vi "Path Is Funnel.vi"(1 "Path Information":T2) -> (0 "Is Funnel?":bool)   [LabVIEW 2013]
doc: "This VI determines whether or not a path is actually a funnel. It must have two curves (C's) and if it has a line (L), the last point must be the same as the starting point."
uses:
  <vilib>/Analysis/Matrix/Datatypes/RealMatrix.ctl
  <vilib>/Analysis/Matrix/NI_Matrix.lvlib
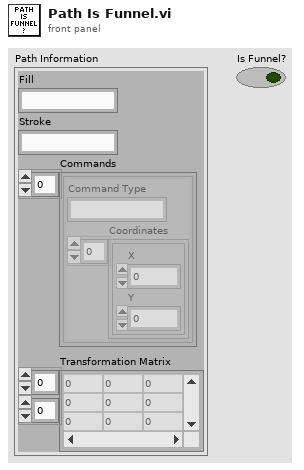
[diagram p1: front panel]
types:
  T1 = typedef "NI_Matrix.lvlib/RealMatrix.ctl" = dbl[][]
  T2 = cluster{"Fill":string, "Stroke":string, "Commands":cluster{"Command Type":string, "Coordinates":cluster{"X":dbl, "Y":dbl}[]}[], "Transformation Matrix":T1}
  T3 = cluster{"Command Type":string, "Coordinates":cluster{"X":dbl, "Y":dbl}[]}[]
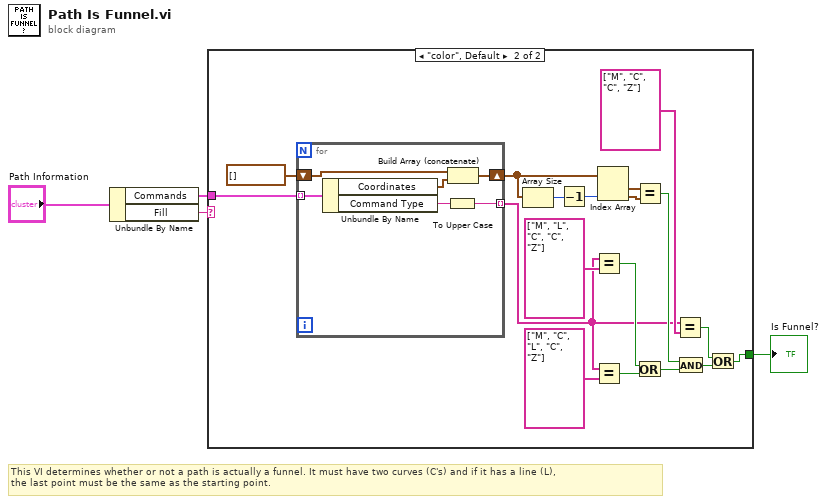
[diagram p0: block diagram]
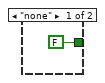
[diagram p2: hidden frame]
diagram:
  # "This VI determines whether or not a path is actually a funnel. It must have two curves (C's) and if it has a line (L),\nthe last point must be the same as the starting point."
  n1 = Unbundle By Name("Path Information") -> ("Commands"=w3:T3, "Fill"=w4:string)
  n2 = case shown="\"color\", Default" w4 {
    tunnel: w3 -> [_ w7]
    tunnel: [FALSE w6] -> w1
    frame "none" {
    }
    frame "color", Default {
      n3 = for {
        tunnel: w7 -> [w29] mode=indexing
        tunnel: [w24] -> w8 mode=indexing
        shift-right: [w27] -> w13
        shift-left: cluster{"X":dbl, "Y":dbl}[] [] -> [w28]
        n4 = Unbundle By Name(w29) -> ("Coordinates"=w26:cluster{"X":dbl, "Y":dbl}[], "Command Type"=w25:string)
        n5 = To Upper Case(1:w25) -> (0:w24:string)
        n6 = Build Array (concatenate)(w28, w26) -> (w27:cluster{"X":dbl, "Y":dbl}[])
      }
      n7 = Array Size(array=w13) -> (size(s)=w12:i32)
      n8 = Decrement(x=w12) -> (x-1=w11:i32)
      n9 = Equal?(x=w8, y=string[] ["M", "L", "C", "C", "Z"]) -> (x = y?=w15:bool)
      n10 = Equal?(x=w8, y=string[] ["M", "C", "L", "C", "Z"]) -> (x = y?=w14:bool)
      n11 = Index Array(array=w13, index #2=w11) -> (element #1=w19:cluster{"X":dbl, "Y":dbl}, element #2=w20:cluster{"X":dbl, "Y":dbl})  [unwired: 1 in]
      n12 = Equal?(x=w19, y=w20) -> (x = y?=w21:bool)
      n13 = Or(x=w15, y=w14) -> (x .or. y?=w18:bool)
      n14 = Equal?(x=w8, y=string[] ["M", "C", "C", "Z"]) -> (x = y?=w23:bool)
      n15 = And(x=w21, y=w18) -> (x .and. y?=w22:bool)
      n16 = Or(x=w23, y=w22) -> (x .or. y?=w6:bool)
    }
  }
  "Is Funnel?" <- w1
